vi "Create All Message Queues.vi"(8 "error in (no error)":errorcluster) -> (0 "error out":errorcluster, 3 "Message Queues out":T1)   [LabVIEW 2022 SP3, in "Message Queue.lvlib"]
doc: "This VI creates and initializes all the message queues for your application. If your application requires more than one message queue, right-click the \"Message Queues\" constant above and select Open Type Def. Add the new Message Queue(s) to the type definition, then initialize them in this VI."
uses:
  Message Queue.lvlib
  Message Cluster.ctl
  Enqueue Message (Single).vi
  All Message Queues.ctl
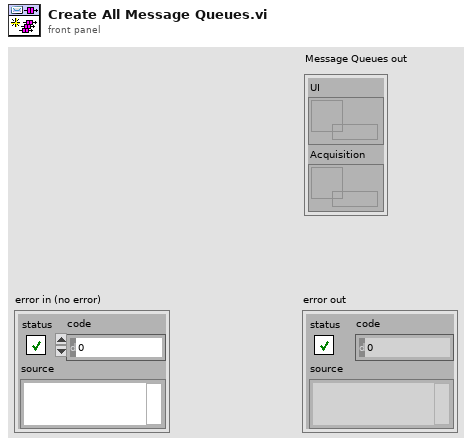
[diagram p1: front panel]
types:
  T1 = cluster{"UI":refnum<queue>, "Acquisition":refnum<queue>}
  T2 = typedef "Message Queue.lvlib/All Message Queues.ctl" = cluster{"UI":refnum<queue>, "Acquisition":refnum<queue>}
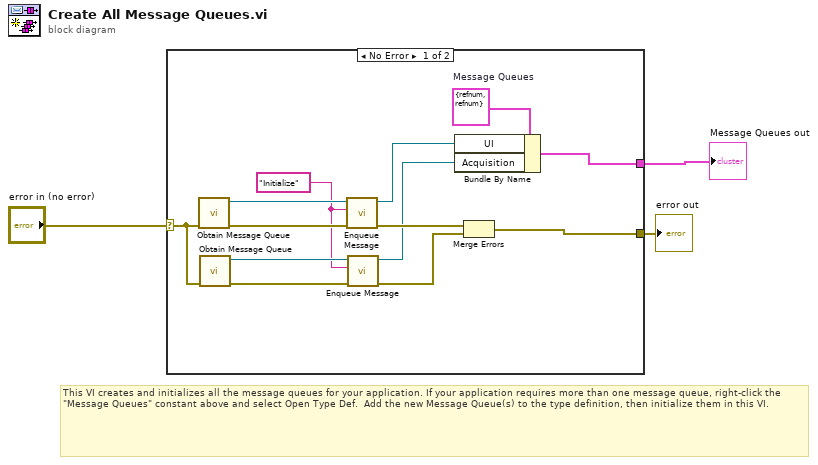
[diagram p0: block diagram]
diagram:
  # "This VI creates and initializes all the message queues for your application. If your application requires more than one message queue, right-click the \"Message Queues\" constant above and select Open Type Def.  Add the new Message Queue(s) to the type definition, then initialize them in this VI."
  n1 = case shown="No Error" "error in (no error)" {
    selector: "error in (no error)" -> [w9 w17]
    tunnel: [w5 w17] -> w3
    tunnel: [w14 _] -> w2
    frame No Error {
      w8 = "Initialize" ("Message")
      w15 = T2 {"UI"=refnum, "Acquisition"=refnum}  # Message Queues
      n2 = call "Obtain Message Queue.vi"("error in (no error)"=w9) -> ("error out"=w13:errorcluster, "Message Queue"=w12:refnum<queue>)  [unwired: 9 in]
      n3 = call "Obtain Message Queue.vi"("error in (no error)"=w9) -> ("error out"=w10:errorcluster, "Message Queue"=w11:refnum<queue>)  [unwired: 9 in]
      n4 = call-poly "Enqueue Message.vi"("error in (no error)"=w13, "Message"=w8, "Message Queue"=w12) -> ("error out"=w16:errorcluster, "dup Message Queue"=w7:refnum<queue>)  [unwired: 7 in]
      n5 = call-poly "Enqueue Message.vi"("error in (no error)"=w10, "Message"=w8, "Message Queue"=w11) -> ("error out"=w4:errorcluster, "dup Message Queue"=w6:refnum<queue>)  [unwired: 7 in]
      n6 = Bundle By Name(cluster=w15, "UI"=w7, "Acquisition"=w6) -> (w14:T2)
      n7 = Merge Errors(w16, w4) -> (w5:errorcluster)
    }
    frame Error {
    }
  }
  "Message Queues out" <- w2
  "error out" <- w3
